vi "Filter SRs.vi"(8 "error in":errorcluster, 9 "Filter Cluster":T1={"Show Resolved"=TRUE, "Show Potentially Resolved"=TRUE, "Show Passoffs"=TRUE, "Show In Collab"=TRUE}, 11 "list in":T2[](array[typedef]) {"Creation Date" format="%<%x>T"; "Last Updated" format="%<%x>T"}) -> (0 "error out":errorcluster, 3 "list out":T2[](array[typedef]) {"Creation Date" format="%<%x>T"; "Last Updated" format="%<%x>T"})   [LabVIEW 2018]
uses:
  Type Defs/SR Cluster.ctl
  Type Defs/SR Status.ctl
  Type Defs/Filter Cluster.ctl
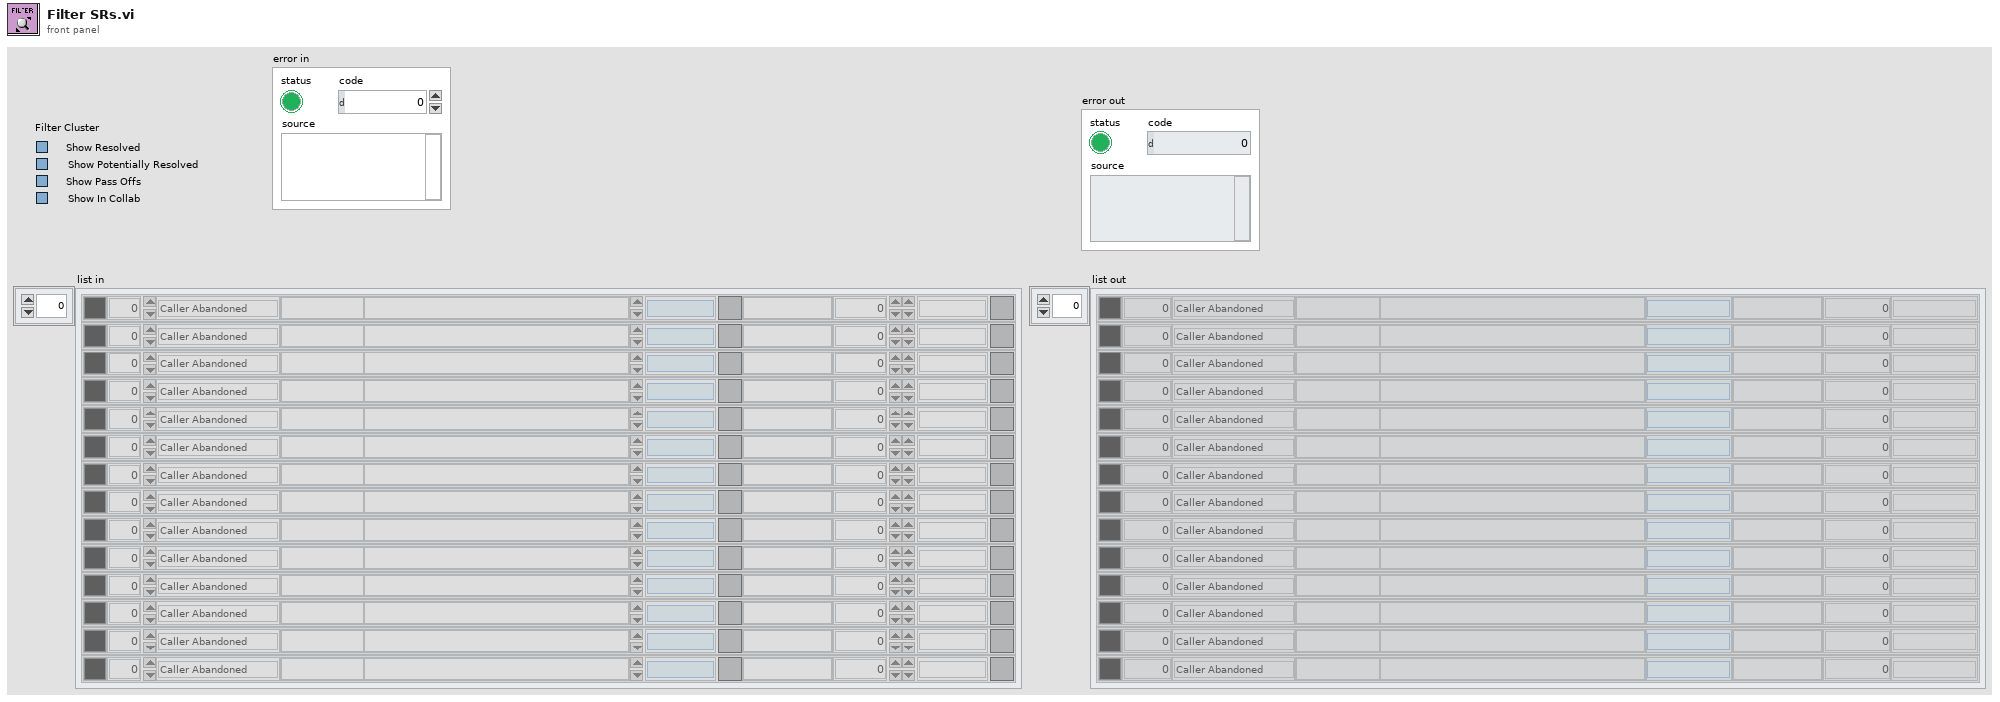
[diagram p1: front panel]
types:
  T1 = typedef "Filter Cluster.ctl" = cluster{"Show Resolved":bool, "Show Potentially Resolved":bool, "Show Passoffs":bool, "Show In Collab":bool}
  T2 = typedef "SR Cluster.ctl" = cluster{"Color":u32, "SR Number":i32, "SR Status":T3, "SR Type":string, "Summary":string, "Last Updated":timestamp, "Service Level":string, "Days Open":dbl, "Creation Date":timestamp}
  T3 = typedef "SR Status.ctl" = enum16{"Caller Abandoned", "Created in Error", "Expired", "Forum Resolved AE", "Forum Resolved Customer", "IN WORK", "IN WORK Collab with AES", "IN WORK Collab with PSE", "IN WORK Collab with SE", "IN WORK Customer Added Note", "IN WORK Escalation", "IN WORK Wait on Customer", "Open", "Potentially Resolved", "Presumed Resolved", "RMA Approved for Return", "Resolved", "Passed Off"}
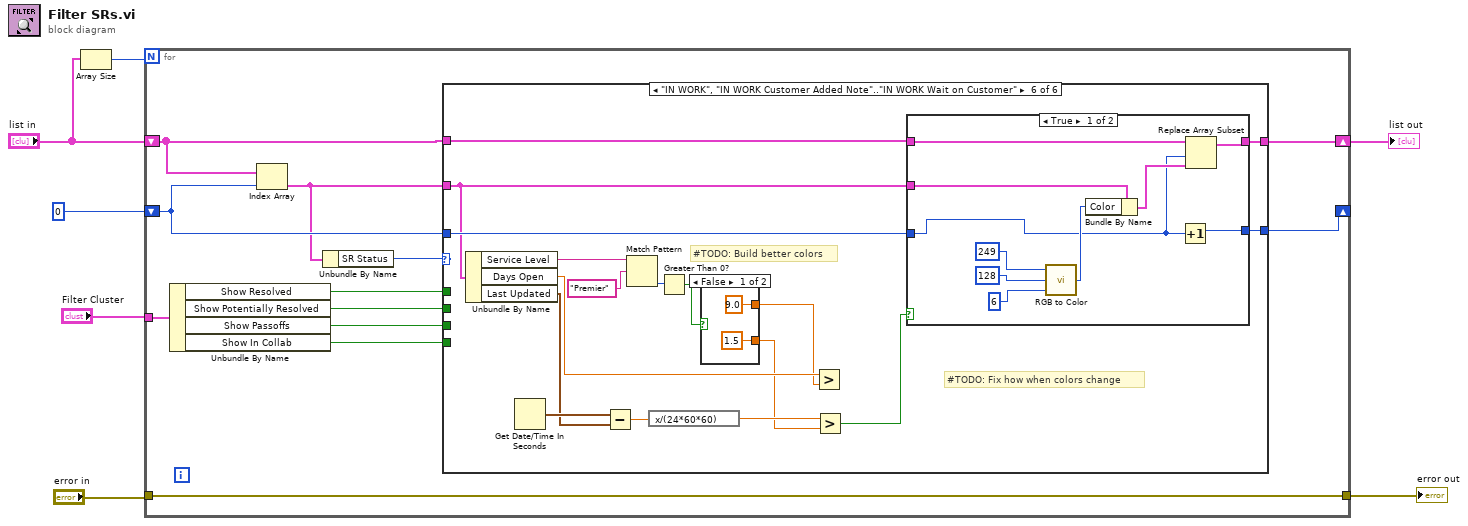
[diagram p0: block diagram]
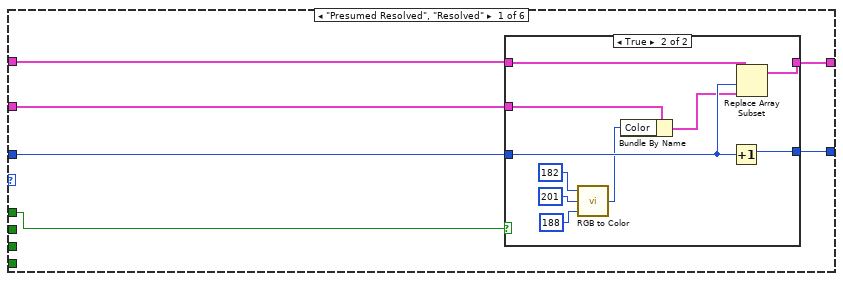
[diagram p2: hidden frame]
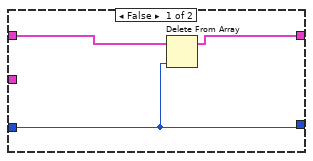
[diagram p3: hidden frame]
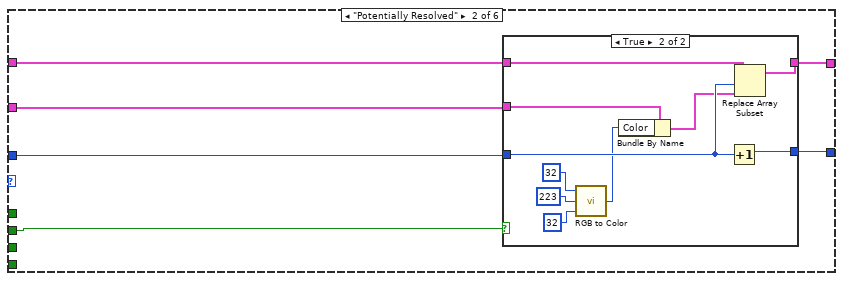
[diagram p4: hidden frame]
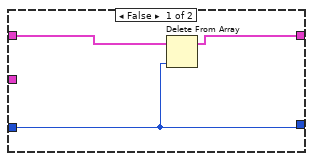
[diagram p5: hidden frame]
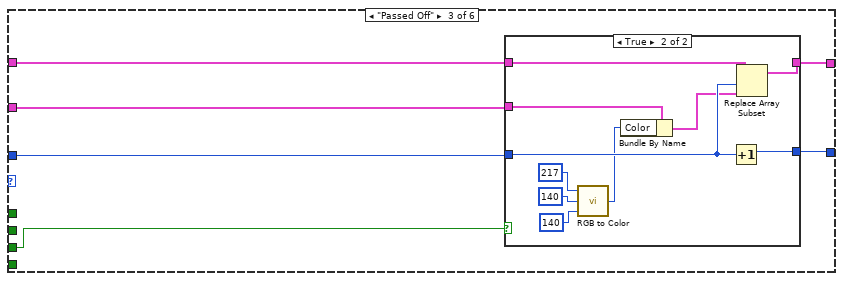
[diagram p6: hidden frame]
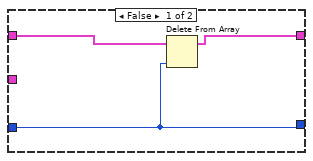
[diagram p7: hidden frame]
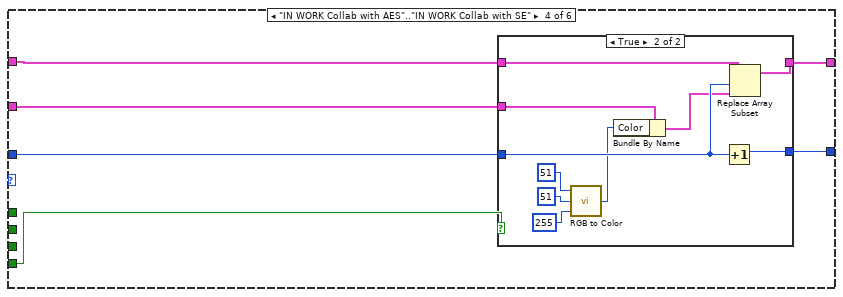
[diagram p8: hidden frame]
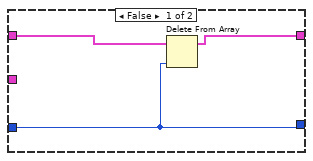
[diagram p9: hidden frame]
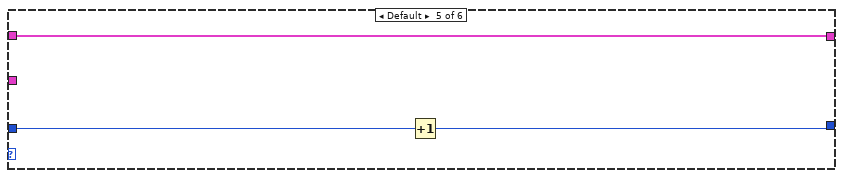
[diagram p10: hidden frame]
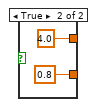
[diagram p11: hidden frame]
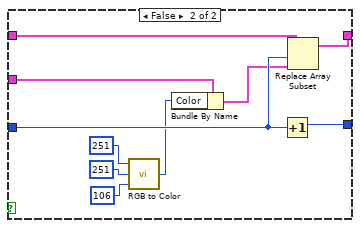
[diagram p12: hidden frame]
diagram:
  n1 = Array Size(array="list in") -> (size(s)=w6:i32)
  n2 = for {
    N: w6 -> [_]
    tunnel: "Filter Cluster" -> [w8]
    shift-right: [w12] -> w7
    shift-left: "list in" -> [w13]
    shift-right: [w14] -> _
    shift-left: 0 -> [w11]
    tunnel: "error in" -> [w10]
    tunnel: [w10] -> w3
    n3 = Unbundle By Name(w8) -> ("Show Resolved"=w18:bool, "Show Potentially Resolved"=w17:bool, "Show Passoffs"=w16:bool, "Show In Collab"=w15:bool)
    n4 = Index Array(array=w13, index=w11) -> (element=w9:T2)
    n5 = Unbundle By Name(w9) -> ("SR Status"=w19:T3)
    n6 = case shown="\"IN WORK\", \"IN WORK Customer Added Note\"..\"IN WORK Wait on Customer\"" w19 {
      tunnel: w18 -> [w25 _ _ _ _ _]
      tunnel: w17 -> [_ w41 _ _ _ _]
      tunnel: w16 -> [_ _ w58 _ _ _]
      tunnel: w15 -> [_ _ _ w78 _ _]
      tunnel: w11 -> [w24 w42 w61 w82 w97 w114]
      tunnel: [w20 w40 w60 w81 w96 w113] -> w14
      tunnel: w13 -> [w22 w44 w63 w80 w98 w115]
      tunnel: [w21 w39 w59 w79 w98 w112] -> w12
      tunnel: w9 -> [w23 w43 w62 w77 _ w111]
      frame "Presumed Resolved", "Resolved" {
        n7 = case shown="True" w25 {
          tunnel: w24 -> [w26 w37]
          tunnel: [w26 w38] -> w20
          tunnel: w22 -> [w28 w36]
          tunnel: [w27 w35] -> w21
          tunnel: w23 -> [_ w34]
          frame False {
            n8 = Delete From Array(array=w28, index=w26) -> (array with subset deleted=w27:T2[])  [unwired: 1 in, 1 out]
          }
          frame True {
            n9 = call <vilib>:"RGB to Color.vi"("B"=u8 188, "G"=u8 201, "R"=u8 182) -> ("Color"=w32:u32)
            n10 = Bundle By Name(cluster=w34, "Color"=w32) -> (w33:T2)
            n11 = Increment(x=w37) -> (x+1=w38:i32)
            n12 = Replace Array Subset(array=w36, new element=w33, index=w37) -> (w35:T2[])
          }
        }
      }
      frame "Potentially Resolved" {
        n13 = case shown="True" w41 {
          tunnel: w42 -> [w45 w56]
          tunnel: [w45 w57] -> w40
          tunnel: w44 -> [w47 w55]
          tunnel: [w46 w54] -> w39
          tunnel: w43 -> [_ w53]
          frame False {
            n14 = Delete From Array(array=w47, index=w45) -> (array with subset deleted=w46:T2[])  [unwired: 1 in, 1 out]
          }
          frame True {
            n15 = call <vilib>:"RGB to Color.vi"("B"=u8 32, "G"=u8 223, "R"=u8 32) -> ("Color"=w51:u32)
            n16 = Bundle By Name(cluster=w53, "Color"=w51) -> (w52:T2)
            n17 = Increment(x=w56) -> (x+1=w57:i32)
            n18 = Replace Array Subset(array=w55, new element=w52, index=w56) -> (w54:T2[])
          }
        }
      }
      frame "Passed Off" {
        n19 = case shown="True" w58 {
          tunnel: w61 -> [w64 w75]
          tunnel: [w64 w76] -> w60
          tunnel: w63 -> [w66 w74]
          tunnel: [w65 w73] -> w59
          tunnel: w62 -> [_ w72]
          frame False {
            n20 = Delete From Array(array=w66, index=w64) -> (array with subset deleted=w65:T2[])  [unwired: 1 in, 1 out]
          }
          frame True {
            n21 = call <vilib>:"RGB to Color.vi"("B"=u8 140, "G"=u8 140, "R"=u8 217) -> ("Color"=w70:u32)
            n22 = Bundle By Name(cluster=w72, "Color"=w70) -> (w71:T2)
            n23 = Increment(x=w75) -> (x+1=w76:i32)
            n24 = Replace Array Subset(array=w74, new element=w71, index=w75) -> (w73:T2[])
          }
        }
      }
      frame "IN WORK Collab with AES".."IN WORK Collab with SE" {
        n25 = case shown="True" w78 {
          tunnel: w82 -> [w83 w94]
          tunnel: [w83 w95] -> w81
          tunnel: w80 -> [w85 w93]
          tunnel: [w84 w92] -> w79
          tunnel: w77 -> [_ w91]
          frame False {
            n26 = Delete From Array(array=w85, index=w83) -> (array with subset deleted=w84:T2[])  [unwired: 1 in, 1 out]
          }
          frame True {
            n27 = call <vilib>:"RGB to Color.vi"("B"=u8 255, "G"=u8 51, "R"=u8 51) -> ("Color"=w89:u32)
            n28 = Bundle By Name(cluster=w91, "Color"=w89) -> (w90:T2)
            n29 = Increment(x=w94) -> (x+1=w95:i32)
            n30 = Replace Array Subset(array=w93, new element=w90, index=w94) -> (w92:T2[])
          }
        }
      }
      frame Default {
        n31 = Increment(x=w97) -> (x+1=w96:i32)
      }
      frame "IN WORK", "IN WORK Customer Added Note".."IN WORK Wait on Customer" {
        # "#TODO: Fix how when colors change"
        # "#TODO: Build better colors"
        n32 = Unbundle By Name(w111) -> ("Service Level"=w110:string, "Days Open"=w106:dbl, "Last Updated"=w104:timestamp)
        n33 = Get Date/Time In Seconds() -> (seconds since 1Jan1904=w105:timestamp)
        n34 = Subtract(x=w105, y=w104) -> (x-y=w103:dbl)
        n35 = Match Pattern(string=w110, regular expression="Premier") -> (offset past match=w109:i32)  [unwired: 1 in, 3 out]
        n36 = expression code="x/(24*60*60)"(w103) -> (w102:dbl)
        n37 = Greater Than 0?(x=w109) -> (x > 0?=w107:bool)
        n38 = case shown="False" w107 {
          tunnel: [1.5 ("y") 0.8 ("y")] -> w101
          tunnel: [9.0 ("y") 4.0 ("y")] -> w100
          frame False {
          }
          frame True {
          }
        }
        n39 = Greater?(x=w106, y=w100) -> ()  [unwired: 1 out]
        n40 = Greater?(x=w102, y=w101) -> (0:w99:bool)
        n41 = case shown="True" w99 {
          tunnel: w114 -> [w120 w138]
          tunnel: [w129 w139] -> w113
          tunnel: w115 -> [w128 w137]
          tunnel: [w127 w136] -> w112
          tunnel: w111 -> [w126 w135]
          frame True {
            n42 = call <vilib>:"RGB to Color.vi"("B"=u8 6, "G"=u8 128, "R"=u8 249) -> ("Color"=w124:u32)
            n43 = Bundle By Name(cluster=w126, "Color"=w124) -> (w125:T2)
            n44 = Increment(x=w120) -> (x+1=w129:i32)
            n45 = Replace Array Subset(array=w128, new element=w125, index=w120) -> (w127:T2[])
          }
          frame False {
            n46 = call <vilib>:"RGB to Color.vi"("B"=u8 106, "G"=u8 251, "R"=u8 251) -> ("Color"=w133:u32)
            n47 = Bundle By Name(cluster=w135, "Color"=w133) -> (w134:T2)
            n48 = Increment(x=w138) -> (x+1=w139:i32)
            n49 = Replace Array Subset(array=w137, new element=w134, index=w138) -> (w136:T2[])
          }
        }
      }
    }
  }
  "error out" <- w3
  "list out" <- w7
